vi "Get Path to Plugin UI.vi"(8 "error in (no error)":errorcluster, 11 "Plugin Info":T1 {"Node Status"."Monitor Doubles"."4" format="%#_9g"; "Node Status"."Monitor Doubles"."3" format="%#_9g"; "Node Status"."Monitor Doubles"."2" format="%#_9g"; "Node Status"."Monitor Doubles"."1" format="%#_9g"; "Node Status"."Timing Statistics (us)"."Period"."Avg" format="%_6g"}) -> (0 "error out":errorcluster, 3 "Plugin UI Path":path)   [LabVIEW 2021, in "CIF_UI.lvclass"]
uses:
  CIF_UI.lvclass
  Typedef/PluginInfo.ctl
  Typedef/Version.ctl
  CIFCore/Common/Typedef/gRPC Reported Plugin Status.ctl
  CIFCore/Common/Typedef/Plugin State.ctl
  CIFCore/Common/Typedef/Timing Statistics.ctl
  CIFCore/Common/Typedef/Timing Stats Base.ctl
  CIFCore/Common/Typedef/FIFO Statistics.ctl
  CIFCore/Common/Typedef/Simple Error.ctl
  CIFCore/Common/Typedef/Monitor Doubles.ctl
  CIFCore/Common/Typedef/Monitor U64.ctl
  CIFCore/Common/Typedef/Monitor I64.ctl
  CIFCore/Common/Typedef/Errors.ctl
  <vilib>/CIF Foundation/CIF Utilities/Errors/Append Error Location.vi
  CIFUtilities/CIFConfigurationFile/CIF Configuration File.lvlib
  CIFCore/Common/CIFCoreCommon.lvlib
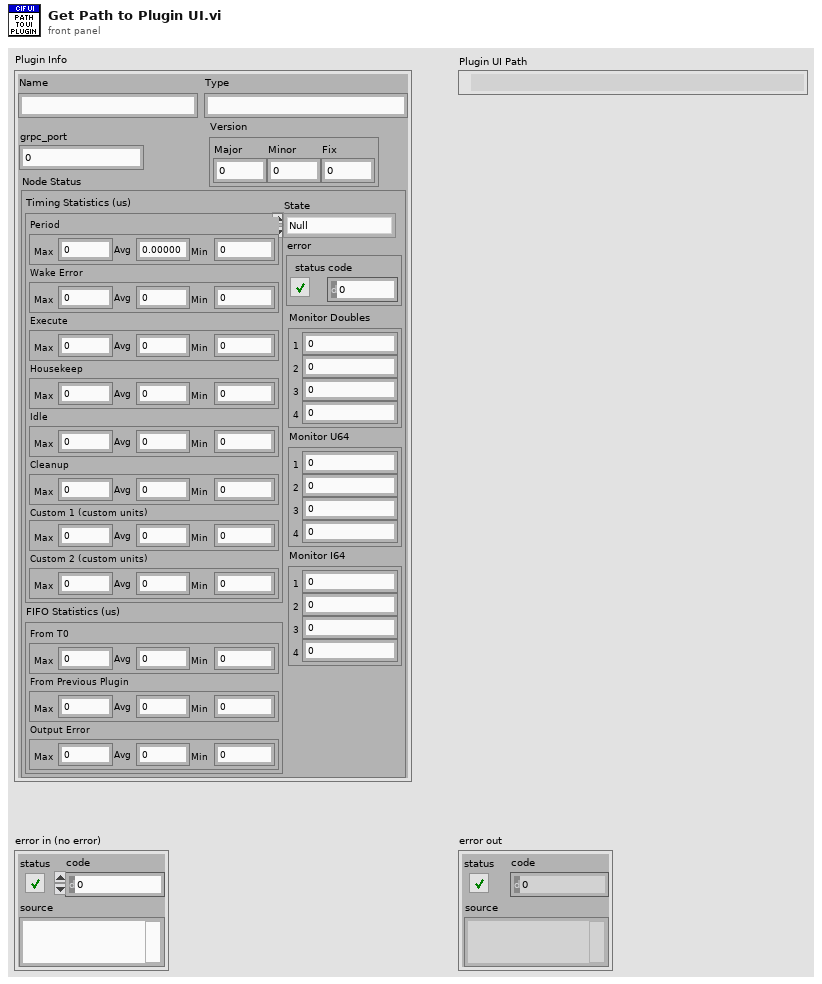
[diagram p1: front panel]
types:
  T1 = typedef "CIF_UI.lvclass/PluginInfo.ctl" = cluster{"Name":string, "Type":string, "grpc_port":i32, "Version":T2, "Node Status":T3}
  T2 = typedef "CIF_UI.lvclass/Version.ctl" = cluster{"Major":i32, "Minor":i32, "Fix":i32}
  T3 = typedef "CIFCoreCommon.lvlib/gRPC Reported Plugin Status.ctl" = cluster{"State":T4, "Timing Statistics (us)":T5, "FIFO Statistics (us)":T7, "error":T8, "Monitor Doubles":T9, "Monitor U64":T10, "Monitor I64":T11}
  T4 = typedef "CIFCoreCommon.lvlib/Plugin State.ctl" = enum32{"Null", "Creating", "Listening", "Running", "CleaningUp", "Destroying"}
  T5 = typedef "CIFCoreCommon.lvlib/Timing Statistics.ctl" = cluster{"Period":T6, "Wake Error":T6, "Execute":T6, "Housekeep":T6, "Idle":T6, "Cleanup":T6, "Custom 1 (custom units)":T6, "Custom 2 (custom units)":T6}
  T6 = typedef "CIFCoreCommon.lvlib/Timing Stats Base.ctl" = cluster{"Max":i64, "Avg":dbl, "Min":i64}
  T7 = typedef "CIFCoreCommon.lvlib/FIFO Statistics.ctl" = cluster{"From T0":T6, "From Previous Plugin":T6, "Output Error":T6}
  T8 = typedef "CIFCoreCommon.lvlib/Simple Error.ctl" = cluster{"status":bool, "code":i32}
  T9 = typedef "CIFCoreCommon.lvlib/Monitor Doubles.ctl" = cluster{"1":dbl, "2":dbl, "3":dbl, "4":dbl}
  T10 = typedef "CIFCoreCommon.lvlib/Monitor U64.ctl" = cluster{"1":u64, "2":u64, "3":u64, "4":u64}
  T11 = typedef "CIFCoreCommon.lvlib/Monitor I64.ctl" = cluster{"1":i64, "2":i64, "3":i64, "4":i64}
  T12 = typedef "CIFCoreCommon.lvlib/Errors.ctl" = enum16{"Invalid Clock ID", "Long Sleep", "gRPC Server Not Found", "Config Parse", "Timestamp Wrap", "Delayed Execution", "Duplicate Channel", "Missing Channel", "Incorrect Type", "Flatten Error", "Unflatten Data", "Unique Name", "Plugin Not Found", "Plugin Type Not Found", "Plugin Version Not Found", "Manager Not Found", "Numerical Issue", "Time Jump", "Clock ID Match", "Channel Length", "Plugin Connection", "gRPC Server Connection", "PPL Name Match", "Build", "Config Log Parse", "Plugin Load", "UI Subpanel Load", "Python Name", "Invalid Name", "Unable to Change Ch Buffer"}
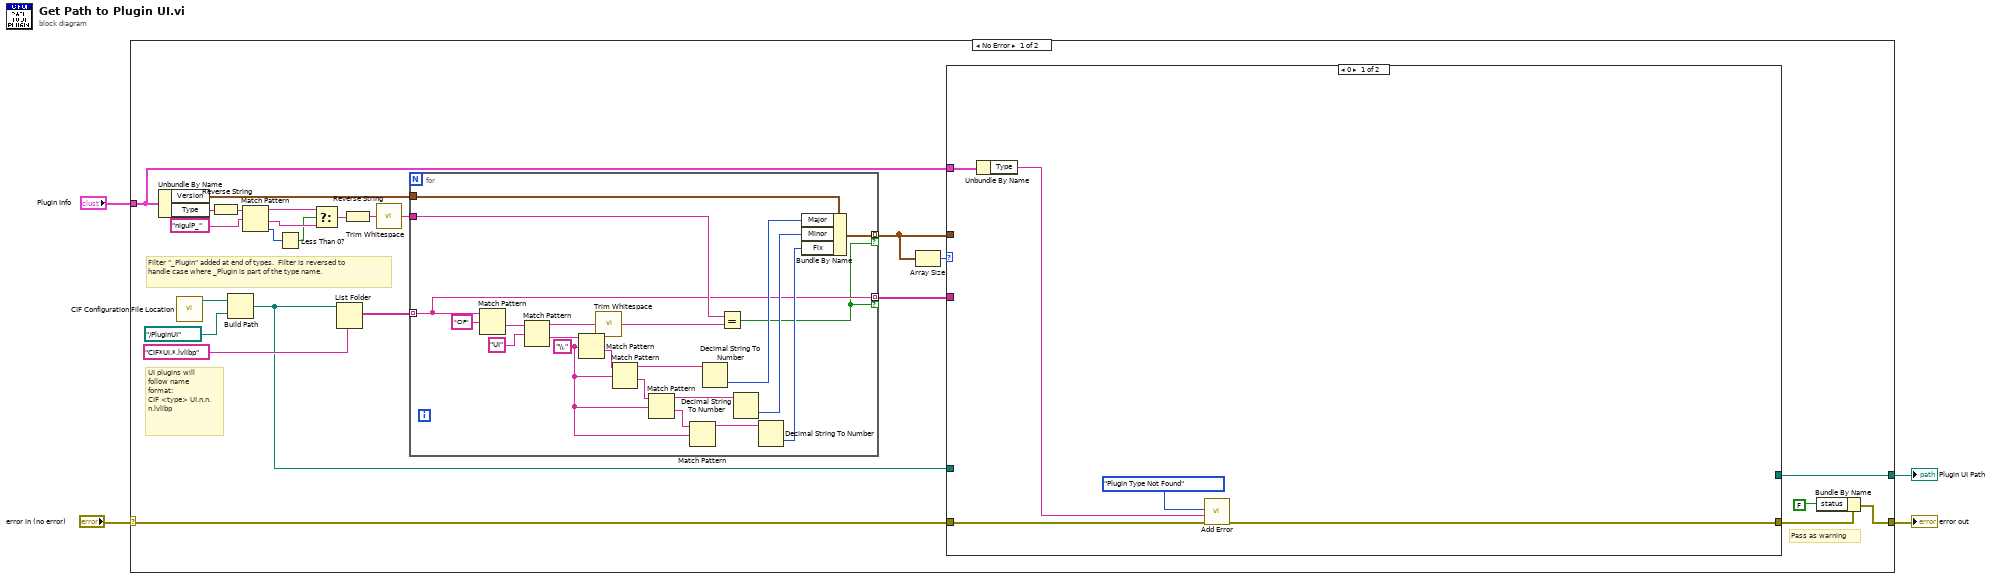
[diagram p0: block diagram]
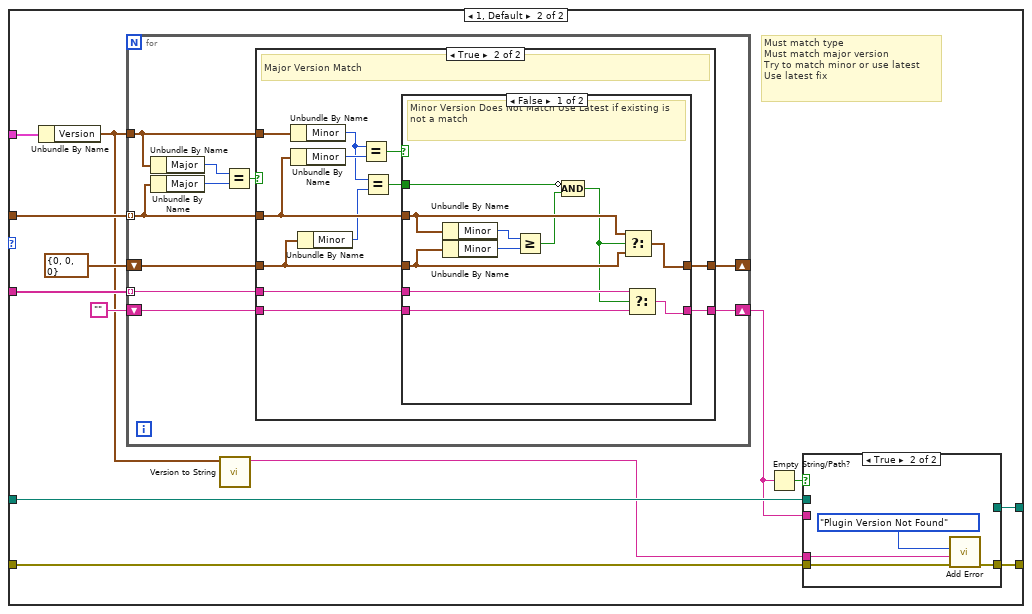
[diagram p2: hidden frame]
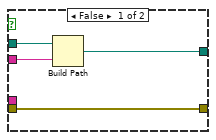
[diagram p3: hidden frame]
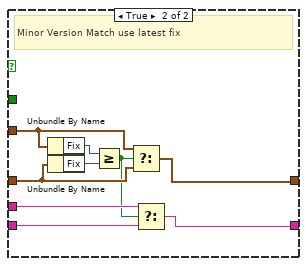
[diagram p5: hidden frame]
diagram:
  n1 = case shown="No Error" "error in (no error)" {
    selector: "error in (no error)" -> [w17 w121]
    tunnel: "Plugin Info" -> [w22 _]
    tunnel: [w14 w121] -> w3
    tunnel: [w18 _] -> w2
    frame No Error {
      # "Filter \"_Plugin\" added at end of types.  Filter is reversed to handle case where _Plugin is part of the type name."
      # "Pass as warning"
      # "UI plugins will follow name format:\nCIF <type> UI.n.n.n.lvlibp"
      n2 = Unbundle By Name(w22) -> ("Version"=w26:T2, "Type"=w12:string)
      n3 = call "CIF Configuration File Location.vi"() -> ("configuration file path"=w29:path)  [unwired: 11 in]
      n4 = Reverse String(1:w12) -> (0:w11:string)
      n5 = Build Path(base path=w29, name or relative path=path "../PluginUI") -> (appended path=w19:path)
      n6 = Match Pattern(string=w11, regular expression="nigulP_") -> (before substring=w9:string, after substring=w7:string, offset past match=w6:i32)  [unwired: 1 in, 1 out]
      n7 = Less Than 0?(x=w6) -> (x < 0?=w5:bool)
      n8 = Select(t=w9, s=w5, f=w7) -> (s? t:f=w8:string)
      n9 = List Folder(path=w19, pattern="CIF*UI.*.lvlibp") -> (filenames=w21:string[])  [unwired: 2 in, 3 out]
      n10 = Reverse String(1:w8) -> (0:w10:string)
      n11 = call <vilib>:"Trim Whitespace.vi"("string"=w10) -> ("trimmed string"=w25:string)  [unwired: 1 in]
      n12 = for {
        tunnel: w21 -> [w101] mode=indexing
        tunnel: w25 -> [w108]
        tunnel: w26 -> [w102]
        tunnel: [w103] -> w24 mode=indexing if=w100
        tunnel: [w101] -> w20 mode=indexing if=w100
        w114 = "\\." ("regular expression")
        n13 = Match Pattern(string=w101, regular expression="CIF") -> (after substring=w119:string)  [unwired: 1 in, 3 out]
        n14 = Match Pattern(string=w119, regular expression="UI") -> (before substring=w116:string, after substring=w117:string)  [unwired: 1 in, 2 out]
        n15 = Match Pattern(string=w117, regular expression=w114) -> (after substring=w115:string)  [unwired: 1 in, 3 out]
        n16 = call <vilib>:"Trim Whitespace.vi"("string"=w116) -> ("trimmed string"=w107:string)  [unwired: 1 in]
        n17 = Match Pattern(string=w115, regular expression=w114) -> (before substring=w109:string, after substring=w112:string)  [unwired: 1 in, 2 out]
        n18 = Match Pattern(string=w112, regular expression=w114) -> (before substring=w110:string, after substring=w113:string)  [unwired: 1 in, 2 out]
        n19 = Match Pattern(string=w113, regular expression=w114) -> (before substring=w111:string)  [unwired: 1 in, 3 out]
        n20 = Decimal String To Number(string=w109) -> (number=w106:i32)  [unwired: 2 in, 1 out]
        n21 = Equal?(x=w108, y=w107) -> (x = y?=w100:bool)
        n22 = Decimal String To Number(string=w110) -> (number=w105:i32)  [unwired: 2 in, 1 out]
        n23 = Decimal String To Number(string=w111) -> (number=w104:i32)  [unwired: 2 in, 1 out]
        n24 = Bundle By Name(cluster=w102, "Major"=w106, "Minor"=w105, "Fix"=w104) -> (w103:T2)
      }
      n25 = Array Size(array=w24) -> (size(s)=w23:i32)
      n26 = case shown="0" w23 {
        tunnel: w24 -> [_ w47]
        tunnel: w17 -> [w33 w38]
        tunnel: w22 -> [w34 w46]
        tunnel: [w32 w37] -> w15
        tunnel: w20 -> [_ w44]
        tunnel: w19 -> [_ w43]
        tunnel: [_ w42] -> w18
        frame 0 {
          n27 = Unbundle By Name(w34) -> ("Type"=w31:string)
          n28 = call "Add Error.vi"("error in (no error)"=w33, "String to Append"=w31, "Error"=Errors."Plugin Type Not Found") -> ("error out"=w32:errorcluster)  [unwired: 8 in]
        }
        frame 1, Default {
          # "Must match type\nMust match major version\nTry to match minor or use latest\nUse latest fix"
          n29 = Unbundle By Name(w46) -> ("Version"=w36:T2)
          n30 = for {
            tunnel: w47 -> [w61] mode=indexing
            tunnel: w36 -> [w62]
            shift-right: [w59] -> _
            shift-left: T2 {"Major"=0, "Minor"=0, "Fix"=0} ("Version") -> [w60]
            tunnel: w44 -> [w58] mode=indexing
            shift-right: [w57] -> w40
            shift-left: "" -> [w56]
            n31 = Unbundle By Name(w62) -> ("Major"=w64:i32)
            n32 = Unbundle By Name(w61) -> ("Major"=w65:i32)
            n33 = Equal?(x=w64, y=w65) -> (x = y?=w63:bool)
            n34 = case shown="True" w63 {
              tunnel: w62 -> [_ w77]
              tunnel: w61 -> [_ w76]
              tunnel: w60 -> [w67 w71]
              tunnel: [w67 w75] -> w59
              tunnel: w58 -> [_ w74]
              tunnel: [w66 w73] -> w57
              tunnel: w56 -> [w66 w72]
              frame False {
                # "Major Version Does Not Match"
              }
              frame True {
                # "Major Version Match"
                n35 = Unbundle By Name(w77) -> ("Minor"=w69:i32)
                n36 = Unbundle By Name(w76) -> ("Minor"=w79:i32)
                n37 = Unbundle By Name(w71) -> ("Minor"=w70:i32)
                n38 = Equal?(x=w69, y=w79) -> (x = y?=w78:bool)
                n39 = Equal?(x=w69, y=w70) -> (x = y?=w68:bool)
                n40 = case shown="False" w78 {
                  tunnel: w76 -> [w90 w99]
                  tunnel: w71 -> [w89 w98]
                  tunnel: [w86 w97] -> w75
                  tunnel: w74 -> [w85 w96]
                  tunnel: [w83 w95] -> w73
                  tunnel: w72 -> [w84 w94]
                  tunnel: w68 -> [w81 _]
                  frame False {
                    # "Minor Version Does Not Match Use Latest if existing is not a match"
                    n41 = Unbundle By Name(w90) -> ("Minor"=w88:i32)
                    n42 = Unbundle By Name(w89) -> ("Minor"=w87:i32)
                    n43 = Greater Or Equal?(x=w88, y=w87) -> (x >= y?=w82:bool)
                    n44 = Compound Arithmetic op=AND(invert w81, w82) -> (w80:bool)
                    n45 = Select(t=w90, s=w80, f=w89) -> (s? t:f=w86:T2)
                    n46 = Select(t=w85, s=w80, f=w84) -> (s? t:f=w83:string)
                  }
                  frame True {
                    # "Minor Version Match use latest fix"
                    n47 = Unbundle By Name(w99) -> ("Fix"=w93:i32)
                    n48 = Unbundle By Name(w98) -> ("Fix"=w92:i32)
                    n49 = Greater Or Equal?(x=w93, y=w92) -> (x >= y?=w91:bool)
                    n50 = Select(t=w99, s=w91, f=w98) -> (s? t:f=w97:T2)
                    n51 = Select(t=w96, s=w91, f=w94) -> (s? t:f=w95:string)
                  }
                }
              }
            }
          }
          n52 = call "Version to String.vi"("Version"=w36) -> ("Version String"=w35:string)  [unwired: 10 in]
          n53 = Empty String/Path?(string/path=w40) -> (empty?=w39:bool)
          n54 = case shown="True" w39 {
            tunnel: w43 -> [w51 _]
            tunnel: w40 -> [w50 _]
            tunnel: [w49 _] -> w42
            tunnel: w38 -> [w48 w54]
            tunnel: [w48 w55] -> w37
            tunnel: w35 -> [_ w53]
            frame False {
              n55 = Build Path(base path=w51, name or relative path=w50) -> (appended path=w49:path)
            }
            frame True {
              n56 = call "Add Error.vi"("error in (no error)"=w54, "String to Append"=w53, "Error"=Errors."Plugin Version Not Found") -> ("error out"=w55:errorcluster)  [unwired: 8 in]
            }
          }
        }
      }
      n57 = Bundle By Name(cluster=w15, "status"=FALSE) -> (w14:errorcluster)
    }
    frame Error {
    }
  }
  "error out" <- w3
  "Plugin UI Path" <- w2
